vi "FreeAnyReference.vi"(8 "error in (no error)":errorcluster, 11 "gRPCid in":T1) -> (0 "error out":errorcluster)   [LabVIEW 2019, in "Template Server.lvlib" / "gprc-lvsupport.lvlib"]
uses:
  gprc-lvsupport.lvlib
  typeDefs/grpcId.ctl
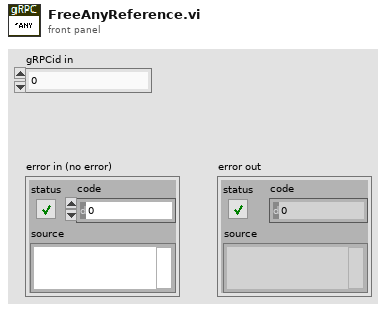
[diagram p1: front panel]
types:
  T1 = typedef "Template Server.lvlib/gprc-lvsupport.lvlib/grpcId.ctl" = u64
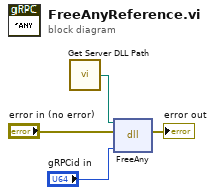
[diagram p0: block diagram]
diagram:
  n1 = call "Get Server DLL Path.vi"() -> ("Server dll path"=w4:path)
  n2 = dll-call lib="?" fn="FreeAny"(path in=w4, error in="error in (no error)", "anyReference"="gRPCid in") -> (error out=→"error out":errorcluster)  [unwired: 3 in, 1 out]
